vi "待签名字符串.vi"(11 "已排序的数组":T1[](array[typedef])) -> (2 "sortQueryString":string, 3 "StringToSign":string)   [LabVIEW 2016]
uses:
  <vilib>/LVH/i3 OAuth/Controls/Name-Value Pair.ctl
  <vilib>/LVH/i3 OAuth/i3-oauth.lvlib
panel:
  in  "HTTPMethod":string(combo)="GET"
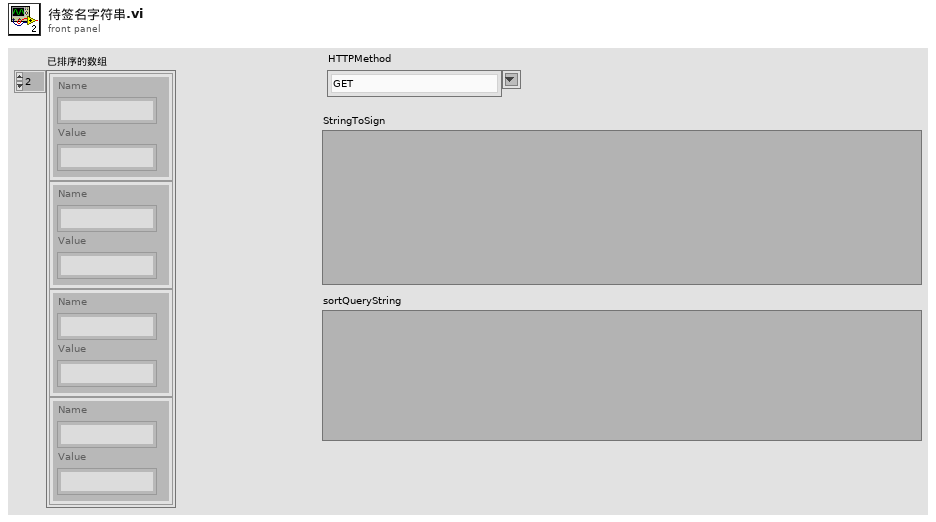
[diagram p1: front panel]
types:
  T1 = typedef "i3-oauth.lvlib/Name-Value Pair.ctl" = cluster{"Name":string, "Value":string}
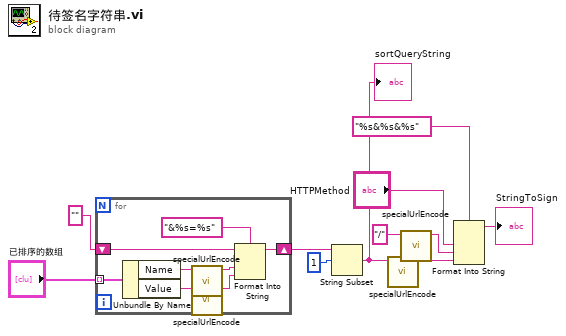
[diagram p0: block diagram]
diagram:
  n1 = for {
    tunnel: "已排序的数组" -> [w17] mode=indexing
    shift-right: [w16] -> w9
    shift-left: "" -> [w19]
    n2 = Unbundle By Name(w17) -> ("Name"=w15:string, "Value"=w13:string)
    n3 = call "specialUrlEncode.vi"("str"=w15) -> ("UrlEncode"=w14:string)  [unwired: 10 in]
    n4 = call "specialUrlEncode.vi"("str"=w13) -> ("UrlEncode"=w12:string)  [unwired: 10 in]
    n5 = Format Into String(format string="&%s=%s" ("格式字符串"), initial string=w19, w14, w12) -> (resulting string=w16:string)  [unwired: 1 in, 1 out]
  }
  n6 = String Subset(string=w9, offset (0)=1 ("偏移量(0)")) -> (substring=w2:string)  [unwired: 1 in]
  "sortQueryString" <- w2
  n7 = call "specialUrlEncode.vi"("str"=w2) -> ("UrlEncode"=w1:string)  [unwired: 10 in]
  n8 = call "specialUrlEncode.vi"("str"="/") -> ("UrlEncode"=w5:string)  [unwired: 10 in]
  n9 = Format Into String(format string="%s&%s&%s" ("格式字符串"), "HTTPMethod", w5, w1) -> (resulting string=→"StringToSign":string)  [unwired: 2 in, 1 out]
